vi "Test Matrix Invert.vi"() -> ()   [LabVIEW 2014, in "Arduino MatrixMath.lvlib"]
uses:
  Arduino MatrixMath.lvlib
panel:
  out "Success?":bool
  out "Error Out":errorcluster
  in  "Error In":errorcluster
  in  "A":sgl[](array[numeric])=[1.0, 2.0, 3.0, 4.0, 5.0, 6.0, 7.0, 8.0]
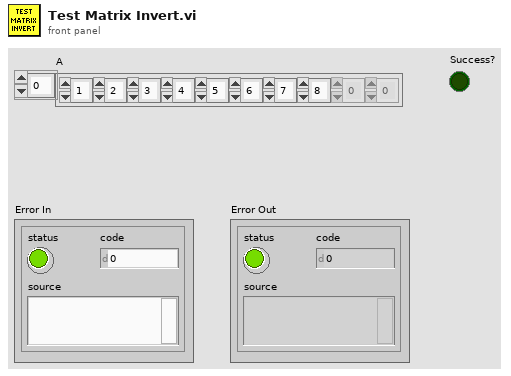
[diagram p1: front panel]
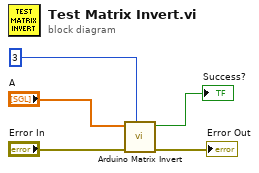
[diagram p0: block diagram]
diagram:
  n1 = call "Arduino Matrix Invert.vi"("rows num. A = (n x n)"=u8 3, "Error In"="Error In", "A"="A") -> ("Error Out"=→"Error Out":errorcluster, "Success?"=→"Success?":bool)  [unwired: 7 in]
